vi "Write instances allowed.vi"(8 "error in":errorcluster, 10 "instances allowed":i32, 11 "decideprojectfeatures in":refnum<class "DecideModuleFeatures.lvclass">) -> (0 "error out":errorcluster, 3 "decideprojectfeatures out":refnum<class "DecideModuleFeatures.lvclass">)   [LabVIEW 2013, in "DecideModuleFeatures.lvclass"]
uses:
  DecideModuleFeatures.lvclass
  DecideModuleFeatures.lvclass/DecideModuleFeatures.ctl
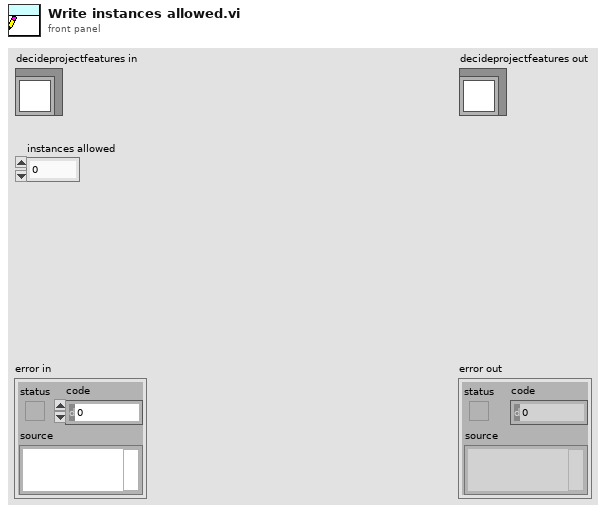
[diagram p1: front panel]
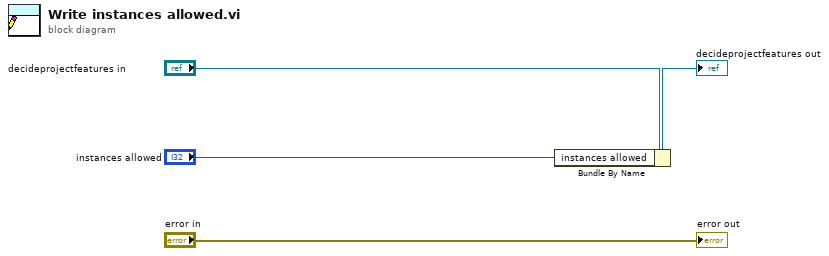
[diagram p0: block diagram]
diagram:
  n1 = Bundle By Name(cluster="decideprojectfeatures in", "instances allowed"="instances allowed") -> (→"decideprojectfeatures out":refnum<class "DecideModuleFeatures.lvclass">)
  "error out" <- "error in"
